vi "Version_2.0_Single_Column_Code.vi"() -> ()   [LabVIEW 2020] (continued)
                                n3037 = call "PortChanger (SubVI).vi"("Port Number"=w3481, "VISA Refnum in"=w3482) -> ()  [unwired: 10 in]
                                }
                                frame #7 {
                                n3038 = local read "VISA Refnum in\nfor Pump"() -> (w3483:refnum<visa-resource-name>)
                                n3039 = call "ProcessCompletionWaiter (SubVI).vi"("VISA Refnum in"=w3483) -> ()  [unwired: 11 in]
                                }
                              }
                            }
                          }
                          frame #3 {
                            # "Wash the pathway between column-2 and column-1 on chip"
                            n3040 = local read "n"() -> (w3484:i32)
                            n3041 = for {
                              N: w3484 -> [_]
                              n3042 = stacked-sequence {
                                frame #0 {
                                n3043 = local read "Buffer-A2 Pumping\nResolution"() -> (w3487:T2)
                                n3044 = local read "VISA Refnum in\nfor Pump"() -> (w3489:refnum<visa-resource-name>)
                                n3045 = local read "V-S"() -> (w3485:dbl)
                                n3046 = local read "Volume of Syringe"() -> (w3488:dbl)
                                n3047 = call "RPickUp(SubVI).vi"("Volume to be picked up"=w3485, "Volume of Syringe"=w3488, "Resolution of PickUP"=w3487, "PickUp Flow Rate (ul/min)"=150.0, "VISA Refnum in"=w3489) -> ()  [unwired: 6 in, 1 out]
                                }
                                frame #1 {
                                n3048 = local read "Stopper that ends \nthe main loops"() -> (w3490:bool)
                                n3049 = local read "VISA Refnum in\nfor Pump"() -> (w3491:refnum<visa-resource-name>)
                                n3050 = case shown="True" w3490 {
                                frame False {
                                }
                                frame True {
                                n3051 = local read "VISA Refnum in\nfor Pump"() -> (w3492:refnum<visa-resource-name>)
                                n3052 = call "HardStopCurrentProcess (SubVI).vi"("VISA Refnum in"=w3492) -> ()  [unwired: 11 in]
                                }
                                }
                                n3053 = call "ProcessCompletionWaiter (SubVI).vi"("VISA Refnum in"=w3491) -> ()  [unwired: 11 in]
                                }
                                frame #2 {
                                # "Switch to Port-10"
                                # "Port-10 of the pump is conncted to column-2"
                                n3054 = local read "VISA Refnum in\nfor Pump"() -> (w3494:refnum<visa-resource-name>)
                                n3055 = call "PortChanger (SubVI).vi"("Port Number"="10", "VISA Refnum in"=w3494) -> ()  [unwired: 10 in]
                                }
                                frame #3 {
                                n3056 = local read "Stopper that ends \nthe main loops"() -> (w3495:bool)
                                n3057 = local read "VISA Refnum in\nfor Pump"() -> (w3496:refnum<visa-resource-name>)
                                n3058 = case shown="True" w3495 {
                                frame False {
                                }
                                frame True {
                                n3059 = local read "VISA Refnum in\nfor Pump"() -> (w3497:refnum<visa-resource-name>)
                                n3060 = call "HardStopCurrentProcess (SubVI).vi"("VISA Refnum in"=w3497) -> ()  [unwired: 11 in]
                                }
                                }
                                n3061 = call "ProcessCompletionWaiter (SubVI).vi"("VISA Refnum in"=w3496) -> ()  [unwired: 11 in]
                                }
                                frame #4 {
                                n3062 = local read "Buffer-A2 Pumping\nResolution"() -> (w3506:T2)
                                n3063 = local read "VISA Refnum in\nfor Pump"() -> (w3508:refnum<visa-resource-name>)
                                n3064 = local read "f"() -> (w3498:dbl)
                                n3065 = local read "Volume of Syringe"() -> (w3507:dbl)
                                n3066 = call "GoToAbsolutePosition(SubVI).vi"("Absolute Volume Position in Syringe (in ul)"=0.0 ("Volume to be Dispensed"), "Volume of Syringe"=w3507, "Resolution of Pumping"=w3506, "Flow Rate (ul/min)"=w3498, "VISA Refnum in"=w3508) -> ()  [unwired: 6 in, 1 out]
                                n3067 = local read "VISA Refnum in\nfor Valve"() -> (w3500:refnum<visa-resource-name>)
                                n3068 = local read "External Valve \nOPEN"() -> (w3499:string)
                                n3069 = local write "Valve V2 Open"(TRUE ("Valve V2 Open")) -> ()
                                n3070 = local write "Valve V1 Open"(FALSE ("Valve V1 Open")) -> ()
                                n3071 = local write "Valve V4 Open"(FALSE ("Valve V4 Open")) -> ()
                                n3072 = local write "Valve V3 Open"(TRUE ("Valve V3 Open")) -> ()
                                n3073 = call "PortChanger_Valve (SubVI).vi"("Port Number"=w3499, "VISA Refnum in"=w3500) -> ()  [unwired: 10 in]
                                }
                                frame #5 {
                                n3074 = local read "VISA Refnum in\nfor Pump"() -> (w3509:refnum<visa-resource-name>)
                                n3075 = call "ProcessCompletionWaiter (SubVI).vi"("VISA Refnum in"=w3509) -> ()  [unwired: 11 in]
                                }
                                frame #6 {
                                # "Change the port back to Buffer-C1"
                                n3076 = local read "VISA Refnum in\nfor Pump"() -> (w3511:refnum<visa-resource-name>)
                                n3077 = local read "Port for \nC1-Equilibriation"() -> (w3510:string)
                                n3078 = call "PortChanger (SubVI).vi"("Port Number"=w3510, "VISA Refnum in"=w3511) -> ()  [unwired: 10 in]
                                }
                                frame #7 {
                                n3079 = local read "VISA Refnum in\nfor Pump"() -> (w3512:refnum<visa-resource-name>)
                                n3080 = call "ProcessCompletionWaiter (SubVI).vi"("VISA Refnum in"=w3512) -> ()  [unwired: 11 in]
                                }
                              }
                            }
                          }
                          frame #4 {
                            # "Washes the SEC column"
                            n3081 = local read "Apparent Volume\nof Syringe"() -> (w3515:dbl)
                            n3082 = local read "c"() -> (w3516:dbl)
                            n3083 = Quotient & Remainder(x=w3516, y=w3515) -> (x-y*floor(x/y)=w3514:dbl, floor(x/y)=w3513:dbl)
                            n3084 = for {
                              N: w3513 -> [_]
                              n3085 = stacked-sequence {
                                frame #0 {
                                n3086 = local read "Buffer-A2 Pumping\nResolution"() -> (w3519:T2)
                                n3087 = local read "VISA Refnum in\nfor Pump"() -> (w3521:refnum<visa-resource-name>)
                                n3088 = local read "Apparent Volume\nof Syringe"() -> (w3517:dbl)
                                n3089 = local read "Volume of Syringe"() -> (w3520:dbl)
                                n3090 = call "RPickUp(SubVI).vi"("Volume to be picked up"=w3517, "Volume of Syringe"=w3520, "Resolution of PickUP"=w3519, "PickUp Flow Rate (ul/min)"=150.0, "VISA Refnum in"=w3521) -> ()  [unwired: 6 in, 1 out]
                                }
                                frame #1 {
                                n3091 = local read "Stopper that ends \nthe main loops"() -> (w3522:bool)
                                n3092 = local read "VISA Refnum in\nfor Pump"() -> (w3523:refnum<visa-resource-name>)
                                n3093 = case shown="True" w3522 {
                                frame False {
                                }
                                frame True {
                                n3094 = local read "VISA Refnum in\nfor Pump"() -> (w3524:refnum<visa-resource-name>)
                                n3095 = call "HardStopCurrentProcess (SubVI).vi"("VISA Refnum in"=w3524) -> ()  [unwired: 11 in]
                                }
                                }
                                n3096 = call "ProcessCompletionWaiter (SubVI).vi"("VISA Refnum in"=w3523) -> ()  [unwired: 11 in]
                                }
                                frame #2 {
                                # "Switch to Port-10"
                                # "Port-10 of the pump is conncted to column-2 of chip"
                                n3097 = local read "VISA Refnum in\nfor Pump"() -> (w3526:refnum<visa-resource-name>)
                                n3098 = call "PortChanger (SubVI).vi"("Port Number"="10", "VISA Refnum in"=w3526) -> ()  [unwired: 10 in]
                                }
                                frame #3 {
                                n3099 = local read "Stopper that ends \nthe main loops"() -> (w3527:bool)
                                n3100 = local read "VISA Refnum in\nfor Pump"() -> (w3528:refnum<visa-resource-name>)
                                n3101 = case shown="True" w3527 {
                                frame False {
                                }
                                frame True {
                                n3102 = local read "VISA Refnum in\nfor Pump"() -> (w3529:refnum<visa-resource-name>)
                                n3103 = call "HardStopCurrentProcess (SubVI).vi"("VISA Refnum in"=w3529) -> ()  [unwired: 11 in]
                                }
                                }
                                n3104 = call "ProcessCompletionWaiter (SubVI).vi"("VISA Refnum in"=w3528) -> ()  [unwired: 11 in]
                                }
                                frame #4 {
                                # "Keeps the AMF valve after column-1 open and valve after column-2 closed"
                                n3105 = local read "Buffer-A2 Pumping\nResolution"() -> (w3541:T2)
                                n3106 = local read "VISA Refnum in\nfor Pump"() -> (w3543:refnum<visa-resource-name>)
                                n3107 = local read "f"() -> (w3533:dbl)
                                n3108 = local write "Valve V3 Open"(FALSE ("Valve V3 Open")) -> ()
                                n3109 = local write "Valve V2 Open"(FALSE ("Valve V2 Open")) -> ()
                                n3110 = local write "Valve V4 Open"(TRUE ("Valve V4 Open")) -> ()
                                n3111 = local write "Valve V1 Open"(FALSE ("Valve V1 Open")) -> ()
                                n3112 = local read "Volume of Syringe"() -> (w3542:dbl)
                                n3113 = call "GoToAbsolutePosition(SubVI).vi"("Absolute Volume Position in Syringe (in ul)"=0.0 ("Volume to be Dispensed"), "Volume of Syringe"=w3542, "Resolution of Pumping"=w3541, "Flow Rate (ul/min)"=w3533, "VISA Refnum in"=w3543) -> ()  [unwired: 6 in, 1 out]
                                n3114 = local read "VISA Refnum in\nfor Valve"() -> (w3538:refnum<visa-resource-name>)
                                n3115 = local read "External Valve \nCLOSED"() -> (w3534:string)
                                n3116 = local write "Valve V5 Open"(TRUE ("Valve V5 Open")) -> ()
                                n3117 = local write "Valve V6 Open"(FALSE ("Valve V6 Open")) -> ()
                                n3118 = local write "Valve V7 Open"(TRUE ("Valve V7 Open")) -> ()
                                n3119 = call "PortChanger_Valve (SubVI).vi"("Port Number"=w3534, "VISA Refnum in"=w3538) -> ()  [unwired: 10 in]
                                }
                                frame #5 {
                                n3120 = local read "VISA Refnum in\nfor Pump"() -> (w3544:refnum<visa-resource-name>)
                                n3121 = call "ProcessCompletionWaiter (SubVI).vi"("VISA Refnum in"=w3544) -> ()  [unwired: 11 in]
                                }
                                frame #6 {
                                # "Change the port back to Buffer-C1"
                                n3122 = local read "VISA Refnum in\nfor Pump"() -> (w3546:refnum<visa-resource-name>)
                                n3123 = local read "Port for \nC1-Equilibriation"() -> (w3545:string)
                                n3124 = call "PortChanger (SubVI).vi"("Port Number"=w3545, "VISA Refnum in"=w3546) -> ()  [unwired: 10 in]
                                }
                                frame #7 {
                                n3125 = local read "VISA Refnum in\nfor Pump"() -> (w3547:refnum<visa-resource-name>)
                                n3126 = call "ProcessCompletionWaiter (SubVI).vi"("VISA Refnum in"=w3547) -> ()  [unwired: 11 in]
                                }
                              }
                            }
                            n3127 = local write "Reminder of the \nVolume to be \nPumped"(w3514) -> ()
                          }
                          frame #5 {
                            # "Washes the SEC column"
                            n3128 = stacked-sequence {
                              frame #0 {
                                n3129 = local read "Buffer-A2 Pumping\nResolution"() -> (w3550:T2)
                                n3130 = local read "VISA Refnum in\nfor Pump"() -> (w3552:refnum<visa-resource-name>)
                                n3131 = local read "Reminder of the \nVolume to be \nPumped"() -> (w3548:dbl)
                                n3132 = local read "Volume of Syringe"() -> (w3551:dbl)
                                n3133 = call "RPickUp(SubVI).vi"("Volume to be picked up"=w3548, "Volume of Syringe"=w3551, "Resolution of PickUP"=w3550, "PickUp Flow Rate (ul/min)"=150.0, "VISA Refnum in"=w3552) -> ()  [unwired: 6 in, 1 out]
                              }
                              frame #1 {
                                n3134 = local read "Stopper that ends \nthe main loops"() -> (w3553:bool)
                                n3135 = local read "VISA Refnum in\nfor Pump"() -> (w3554:refnum<visa-resource-name>)
                                n3136 = case shown="True" w3553 {
                                frame False {
                                }
                                frame True {
                                n3137 = local read "VISA Refnum in\nfor Pump"() -> (w3555:refnum<visa-resource-name>)
                                n3138 = call "HardStopCurrentProcess (SubVI).vi"("VISA Refnum in"=w3555) -> ()  [unwired: 11 in]
                                }
                                }
                                n3139 = call "ProcessCompletionWaiter (SubVI).vi"("VISA Refnum in"=w3554) -> ()  [unwired: 11 in]
                              }
                              frame #2 {
                                # "Switch to Port-10"
                                # "Port-10 of the pump is conncted to column-2 of chip"
                                n3140 = local read "VISA Refnum in\nfor Pump"() -> (w3557:refnum<visa-resource-name>)
                                n3141 = call "PortChanger (SubVI).vi"("Port Number"="10", "VISA Refnum in"=w3557) -> ()  [unwired: 10 in]
                              }
                              frame #3 {
                                n3142 = local read "Stopper that ends \nthe main loops"() -> (w3558:bool)
                                n3143 = local read "VISA Refnum in\nfor Pump"() -> (w3559:refnum<visa-resource-name>)
                                n3144 = case shown="True" w3558 {
                                frame False {
                                }
                                frame True {
                                n3145 = local read "VISA Refnum in\nfor Pump"() -> (w3560:refnum<visa-resource-name>)
                                n3146 = call "HardStopCurrentProcess (SubVI).vi"("VISA Refnum in"=w3560) -> ()  [unwired: 11 in]
                                }
                                }
                                n3147 = call "ProcessCompletionWaiter (SubVI).vi"("VISA Refnum in"=w3559) -> ()  [unwired: 11 in]
                              }
                              frame #4 {
                                n3148 = local read "Buffer-A2 Pumping\nResolution"() -> (w3572:T2)
                                n3149 = local read "VISA Refnum in\nfor Pump"() -> (w3574:refnum<visa-resource-name>)
                                n3150 = local read "f"() -> (w3564:dbl)
                                n3151 = local read "Volume of Syringe"() -> (w3573:dbl)
                                n3152 = call "GoToAbsolutePosition(SubVI).vi"("Absolute Volume Position in Syringe (in ul)"=0.0 ("Volume to be Dispensed"), "Volume of Syringe"=w3573, "Resolution of Pumping"=w3572, "Flow Rate (ul/min)"=w3564, "VISA Refnum in"=w3574) -> ()  [unwired: 6 in, 1 out]
                                n3153 = local write "Valve V3 Open"(FALSE ("Valve V3 Open")) -> ()
                                n3154 = local write "Valve V2 Open"(FALSE ("Valve V2 Open")) -> ()
                                n3155 = local write "Valve V1 Open"(FALSE ("Valve V1 Open")) -> ()
                                n3156 = local write "Valve V4 Open"(TRUE ("Valve V4 Open")) -> ()
                                n3157 = local read "VISA Refnum in\nfor Valve"() -> (w3569:refnum<visa-resource-name>)
                                n3158 = local read "External Valve \nCLOSED"() -> (w3565:string)
                                n3159 = local write "Valve V6 Open"(TRUE ("Valve V6 Open")) -> ()
                                n3160 = local write "Valve V5 Open"(TRUE ("Valve V5 Open")) -> ()
                                n3161 = local write "Valve V7 Open"(TRUE ("Valve V7 Open")) -> ()
                                n3162 = call "PortChanger_Valve (SubVI).vi"("Port Number"=w3565, "VISA Refnum in"=w3569) -> ()  [unwired: 10 in]
                              }
                              frame #5 {
                                n3163 = local read "VISA Refnum in\nfor Pump"() -> (w3575:refnum<visa-resource-name>)
                                n3164 = call "ProcessCompletionWaiter (SubVI).vi"("VISA Refnum in"=w3575) -> ()  [unwired: 11 in]
                              }
                            }
                          }
                        }
                        n3165 = local write "Washing Column-1"(FALSE ("Washing Column-1")) -> ()
                        n3166 = local write "Washing Column-2"(TRUE ("Washing Column-2")) -> ()
                      }
                      frame #4 {
                        # "Elute Column-1, Divert Sample into Column-2, Elute column-2 and Divert the sample onto Grid"
                        n3167 = stacked-sequence {
                          frame #0 {
                            # "Switch to Port-7"
                            # "Port-7 of pump is connected to Buffer-B"
                            n3168 = local write "Washing Column-2"(FALSE ("Washing Column-2")) -> ()
                            n3169 = local read "VISA Refnum in\nfor Pump"() -> (w3580:refnum<visa-resource-name>)
                            n3170 = local read "Port for \nB-Elution"() -> (w3578:string)
                            n3171 = local write "Affinity Elution On"(TRUE ("Affinity Elution On")) -> ()
                            n3172 = call "PortChanger (SubVI).vi"("Port Number"=w3578, "VISA Refnum in"=w3580) -> ()  [unwired: 10 in]
                            n3173 = local write "Elution of Column-1"(TRUE ("Elution of Column-1")) -> ()
                          }
                          frame #1 {
                            n3174 = local read "VISA Refnum in\nfor Pump"() -> (w3581:refnum<visa-resource-name>)
                            n3175 = call "ProcessCompletionWaiter (SubVI).vi"("VISA Refnum in"=w3581) -> ()  [unwired: 11 in]
                          }
                          frame #2 {
                            # "If Yes, it will clean the elution buffer from port-5 tubing a bit more"
                            n3176 = local read "Clean the \nBuffer-B tubing"() -> (w3582:bool)
                            n3177 = case shown="True" w3582 {
                              frame False {
                                n3178 = stacked-sequence {
                                frame #0 {
                                n3179 = local read "Buffer-B Pumping\nResolution"() -> (w3585:T2)
                                n3180 = local read "VISA Refnum in\nfor Pump"() -> (w3587:refnum<visa-resource-name>)
                                n3181 = local read "V-S"() -> (w3584:dbl)
                                n3182 = local read "Volume of Syringe"() -> (w3586:dbl)
                                n3183 = call "RPickUp(SubVI).vi"("Volume to be picked up"=w3584, "Volume of Syringe"=w3586, "Resolution of PickUP"=w3585, "PickUp Flow Rate (ul/min)"=150.0, "VISA Refnum in"=w3587) -> ()  [unwired: 6 in, 1 out]
                                }
                                frame #1 {
                                n3184 = local read "Stopper that ends \nthe main loops"() -> (w3588:bool)
                                n3185 = local read "VISA Refnum in\nfor Pump"() -> (w3589:refnum<visa-resource-name>)
                                n3186 = case shown="True" w3588 {
                                frame False {
                                }
                                frame True {
                                n3187 = local read "VISA Refnum in\nfor Pump"() -> (w3590:refnum<visa-resource-name>)
                                n3188 = call "HardStopCurrentProcess (SubVI).vi"("VISA Refnum in"=w3590) -> ()  [unwired: 11 in]
                                }
                                }
                                n3189 = call "ProcessCompletionWaiter (SubVI).vi"("VISA Refnum in"=w3589) -> ()  [unwired: 11 in]
                                }
                                frame #2 {
                                n3190 = local read "VISA Refnum in\nfor Pump"() -> (w3592:refnum<visa-resource-name>)
                                n3191 = call "PortChanger (SubVI).vi"("Port Number"="1", "VISA Refnum in"=w3592) -> ()  [unwired: 10 in]
                                }
                                frame #3 {
                                n3192 = local read "Stopper that ends \nthe main loops"() -> (w3593:bool)
                                n3193 = local read "VISA Refnum in\nfor Pump"() -> (w3594:refnum<visa-resource-name>)
                                n3194 = case shown="True" w3593 {
                                frame False {
                                }
                                frame True {
                                n3195 = local read "VISA Refnum in\nfor Pump"() -> (w3595:refnum<visa-resource-name>)
                                n3196 = call "HardStopCurrentProcess (SubVI).vi"("VISA Refnum in"=w3595) -> ()  [unwired: 11 in]
                                }
                                }
                                n3197 = call "ProcessCompletionWaiter (SubVI).vi"("VISA Refnum in"=w3594) -> ()  [unwired: 11 in]
                                }
                                frame #4 {
                                n3198 = local read "VISA Refnum in\nfor Pump"() -> (w3600:refnum<visa-resource-name>)
                                n3199 = local read "Volume of Syringe"() -> (w3597:dbl)
                                n3200 = call "GoToAbsolutePosition(SubVI).vi"("Absolute Volume Position in Syringe (in ul)"=0.0, "Volume of Syringe"=w3597, "Resolution of Pumping"=T2."Standard Pumping", "Flow Rate (ul/min)"=150.0, "VISA Refnum in"=w3600) -> ()  [unwired: 6 in, 1 out]
                                }
                                frame #5 {
                                n3201 = local read "Stopper that ends \nthe main loops"() -> (w3601:bool)
                                n3202 = local read "VISA Refnum in\nfor Pump"() -> (w3602:refnum<visa-resource-name>)
                                n3203 = case shown="True" w3601 {
                                frame False {
                                }
                                frame True {
                                n3204 = local read "VISA Refnum in\nfor Pump"() -> (w3603:refnum<visa-resource-name>)
                                n3205 = call "HardStopCurrentProcess (SubVI).vi"("VISA Refnum in"=w3603) -> ()  [unwired: 11 in]
                                }
                                }
                                n3206 = call "ProcessCompletionWaiter (SubVI).vi"("VISA Refnum in"=w3602) -> ()  [unwired: 11 in]
                                }
                                }
                              }
                              frame True {
                                n3207 = for {
                                N: 2 -> [_]
                                n3208 = stacked-sequence {
                                frame #0 {
                                n3209 = local read "Buffer-B Pumping\nResolution"() -> (w3607:T2)
                                n3210 = local read "VISA Refnum in\nfor Pump"() -> (w3609:refnum<visa-resource-name>)
                                n3211 = local read "Apparent Volume\nof Syringe"() -> (w3606:dbl)
                                n3212 = local read "Volume of Syringe"() -> (w3608:dbl)
                                n3213 = call "RPickUp(SubVI).vi"("Volume to be picked up"=w3606, "Volume of Syringe"=w3608, "Resolution of PickUP"=w3607, "PickUp Flow Rate (ul/min)"=150.0, "VISA Refnum in"=w3609) -> ()  [unwired: 6 in, 1 out]
                                }
                                frame #1 {
                                n3214 = local read "Stopper that ends \nthe main loops"() -> (w3610:bool)
                                n3215 = local read "VISA Refnum in\nfor Pump"() -> (w3611:refnum<visa-resource-name>)
                                n3216 = case shown="True" w3610 {
                                frame False {
                                }
                                frame True {
                                n3217 = local read "VISA Refnum in\nfor Pump"() -> (w3612:refnum<visa-resource-name>)
                                n3218 = call "HardStopCurrentProcess (SubVI).vi"("VISA Refnum in"=w3612) -> ()  [unwired: 11 in]
                                }
                                }
                                n3219 = call "ProcessCompletionWaiter (SubVI).vi"("VISA Refnum in"=w3611) -> ()  [unwired: 11 in]
                                }
                                frame #2 {
                                n3220 = local read "VISA Refnum in\nfor Pump"() -> (w3614:refnum<visa-resource-name>)
                                n3221 = call "PortChanger (SubVI).vi"("Port Number"="1", "VISA Refnum in"=w3614) -> ()  [unwired: 10 in]
                                }
                                frame #3 {
                                n3222 = local read "Stopper that ends \nthe main loops"() -> (w3615:bool)
                                n3223 = local read "VISA Refnum in\nfor Pump"() -> (w3616:refnum<visa-resource-name>)
                                n3224 = case shown="True" w3615 {
                                frame False {
                                }
                                frame True {
                                n3225 = local read "VISA Refnum in\nfor Pump"() -> (w3617:refnum<visa-resource-name>)
                                n3226 = call "HardStopCurrentProcess (SubVI).vi"("VISA Refnum in"=w3617) -> ()  [unwired: 11 in]
                                }
                                }
                                n3227 = call "ProcessCompletionWaiter (SubVI).vi"("VISA Refnum in"=w3616) -> ()  [unwired: 11 in]
                                }
                                frame #4 {
                                n3228 = local read "VISA Refnum in\nfor Pump"() -> (w3622:refnum<visa-resource-name>)
                                n3229 = local read "Volume of Syringe"() -> (w3619:dbl)
                                n3230 = call "GoToAbsolutePosition(SubVI).vi"("Absolute Volume Position in Syringe (in ul)"=0.0, "Volume of Syringe"=w3619, "Resolution of Pumping"=T2."Standard Pumping", "Flow Rate (ul/min)"=150.0, "VISA Refnum in"=w3622) -> ()  [unwired: 6 in, 1 out]
                                }
                                frame #5 {
                                n3231 = local read "Stopper that ends \nthe main loops"() -> (w3623:bool)
                                n3232 = local read "VISA Refnum in\nfor Pump"() -> (w3624:refnum<visa-resource-name>)
                                n3233 = case shown="True" w3623 {
                                frame False {
                                }
                                frame True {
                                n3234 = local read "VISA Refnum in\nfor Pump"() -> (w3625:refnum<visa-resource-name>)
                                n3235 = call "HardStopCurrentProcess (SubVI).vi"("VISA Refnum in"=w3625) -> ()  [unwired: 11 in]
                                }
                                }
                                n3236 = call "ProcessCompletionWaiter (SubVI).vi"("VISA Refnum in"=w3624) -> ()  [unwired: 11 in]
                                }
                                }
                                }
                              }
                            }
                          }
                          frame #3 {
                            n3237 = local read "VISA Refnum in\nfor Pump"() -> (w3627:refnum<visa-resource-name>)
                            n3238 = local read "Port for \nB-Elution"() -> (w3626:string)
                            n3239 = call "PortChanger (SubVI).vi"("Port Number"=w3626, "VISA Refnum in"=w3627) -> ()  [unwired: 10 in]
                          }
                          frame #4 {
                            n3240 = local read "VISA Refnum in\nfor Pump"() -> (w3628:refnum<visa-resource-name>)
                            n3241 = call "ProcessCompletionWaiter (SubVI).vi"("VISA Refnum in"=w3628) -> ()  [unwired: 11 in]
                          }
                          frame #5 {
                            n3242 = local read "Buffer-B PickUp \nFlow Rate (ul/min)"() -> (w3631:dbl)
                            n3243 = local read "Buffer-B Pumping\nResolution"() -> (w3630:T2)
                            n3244 = local read "VISA Refnum in\nfor Pump"() -> (w3633:refnum<visa-resource-name>)
                            n3245 = local read "Buffer-B Volume \nto be  Pumped"() -> (w3629:dbl)
                            n3246 = local read "Volume of Syringe"() -> (w3632:dbl)
                            n3247 = call "RPickUp(SubVI).vi"("Volume to be picked up"=w3629, "Volume of Syringe"=w3632, "Resolution of PickUP"=w3630, "PickUp Flow Rate (ul/min)"=w3631, "VISA Refnum in"=w3633) -> ()  [unwired: 6 in, 1 out]
                          }
                          frame #6 {
                            n3248 = local read "Stopper that ends \nthe main loops"() -> (w3634:bool)
                            n3249 = local read "VISA Refnum in\nfor Pump"() -> (w3635:refnum<visa-resource-name>)
                            n3250 = case shown="True" w3634 {
                              frame False {
                              }
                              frame True {
                                n3251 = local read "VISA Refnum in\nfor Pump"() -> (w3636:refnum<visa-resource-name>)
                                n3252 = call "HardStopCurrentProcess (SubVI).vi"("VISA Refnum in"=w3636) -> ()  [unwired: 11 in]
                              }
                            }
                            n3253 = call "ProcessCompletionWaiter (SubVI).vi"("VISA Refnum in"=w3635) -> ()  [unwired: 11 in]
                          }
                          frame #7 {
                            # "Reads the initial Plunger Position for computing the volume dispensed"
                            n3254 = local read "VISA Refnum in\nfor Pump"() -> (w3638:refnum<visa-resource-name>)
                            n3255 = call "AbsolutePlungerPosition (SubVI).vi"("VISA Refnum in"=w3638) -> ("Plunger Position"=w3637:i32)  [unwired: 10 in]
                            n3256 = local write "Initial Plunger Position"(w3637) -> ()
                          }
                          frame #8 {
                            # "Switch to Port-2"
                            # "Port-2 of the pump is conncted to column-1 of chip"
                            n3257 = local read "VISA Refnum in\nfor Pump"() -> (w3640:refnum<visa-resource-name>)
                            n3258 = call "PortChanger (SubVI).vi"("Port Number"="2", "VISA Refnum in"=w3640) -> ()  [unwired: 10 in]
                          }
                          frame #9 {
                            n3259 = local read "Stopper that ends \nthe main loops"() -> (w3641:bool)
                            n3260 = local read "VISA Refnum in\nfor Pump"() -> (w3642:refnum<visa-resource-name>)
                            n3261 = case shown="True" w3641 {
                              frame False {
                              }
                              frame True {
                                n3262 = local read "VISA Refnum in\nfor Pump"() -> (w3643:refnum<visa-resource-name>)
                                n3263 = call "HardStopCurrentProcess (SubVI).vi"("VISA Refnum in"=w3643) -> ()  [unwired: 11 in]
                              }
                            }
                            n3264 = call "ProcessCompletionWaiter (SubVI).vi"("VISA Refnum in"=w3642) -> ()  [unwired: 11 in]
                          }
                          frame #10 {
                            # "Keeps the AMF valve after column-1 open and valve after column-2 closed"
                            n3265 = local read "VISA Refnum in\nfor Valve"() -> (w3648:refnum<visa-resource-name>)
                            n3266 = local read "External Valve \nOPEN"() -> (w3647:string)
                            n3267 = call "PortChanger_Valve (SubVI).vi"("Port Number"=w3647, "VISA Refnum in"=w3648) -> ()  [unwired: 10 in]
                            n3268 = local write "Valve V1 Open"(TRUE ("Valve V1 Open")) -> ()
                            n3269 = local write "Valve V2 Open"(TRUE ("Valve V2 Open")) -> ()
                            n3270 = local write "Valve V3 Open"(FALSE ("Valve V3 Open")) -> ()
                            n3271 = local write "Valve V4 Open"(FALSE ("Valve V4 Open")) -> ()
                            n3272 = local write "Valve V6 Open"(FALSE ("Valve V6 Open")) -> ()
                            n3273 = local write "Valve V5 Open"(FALSE ("Valve V5 Open")) -> ()
                            n3274 = local write "Valve V7 Open"(FALSE ("Valve V7 Open")) -> ()
                          }
                          frame #11 {
                            n3275 = local read "Buffer-B Dispense\nFlow Rate (ul/min)"() -> (w3658:dbl)
                            n3276 = local read "Buffer-B Pumping\nResolution"() -> (w3657:T2)
                            n3277 = local read "Initial Plunger Position"() -> (w3654:dbl)
                            n3278 = local read "VISA Refnum in\nfor Pump"() -> (w3660:refnum<visa-resource-name>)
                            n3279 = local read "Volume of Syringe"() -> (w3659:dbl)
                            n3280 = call "GoToAbsolutePosition(SubVI).vi"("Absolute Volume Position in Syringe (in ul)"=0.0 ("Volume to be Dispensed"), "Volume of Syringe"=w3659, "Resolution of Pumping"=w3657, "Flow Rate (ul/min)"=w3658, "VISA Refnum in"=w3660) -> ()  [unwired: 6 in, 1 out]
                            n3281 = local write "Pause Data Collection"(FALSE ("Pause Data Collection")) -> ()
                            n3282 = local write "Vol_now"(0.0 ("Vol_now")) -> ()
                            n3283 = local write "Position\nNow"(w3654) -> ()
                          }
                          frame #12 {
                            n3284 = while {
                              stop <- w3667 stop-if-true
                              n3285 = event shown="[0] \"Pause Elution Value\": Value Change" {
                                selector: _ -> [_ _]
                                dyn-events: _ -> [_ _]
                                timeout: 100 -> [_ _]
                                event "Pause Elution\nValue": Value Change {
                                n3286 = event-data() -> ()  [unwired: 1 in, 6 out]
                                n3287 = stacked-sequence {
                                frame #0 {
                                n3288 = local read "Pause Elution"() -> (w3669:bool)
                                n3289 = case shown="False" w3669 {
                                frame False {
                                n3290 = local write "Pause Elution"(TRUE ("Pause Elution")) -> ()
                                }
                                frame True {
                                n3291 = local write "Pause Elution"(FALSE ("Pause Elution")) -> ()
                                }
                                }
                                }
                                frame #1 {
                                n3292 = local read "Pause Elution"() -> (w3672:bool)
                                n3293 = case shown="False" w3672 {
                                frame False {
                                n3294 = local read "Buffer-B Dispense\nFlow Rate (ul/min)"() -> (w3677:dbl)
                                n3295 = local read "VISA Refnum in\nfor Pump"() -> (w3678:refnum<visa-resource-name>)
                                n3296 = local read "Buffer-B Pumping\nResolution"() -> (w3674:T2)
                                n3297 = local read "Volume of Syringe"() -> (w3675:dbl)
                                n3298 = call "GoToAbsolutePosition(SubVI).vi"("Absolute Volume Position in Syringe (in ul)"=0.0, "Volume of Syringe"=w3675, "Resolution of Pumping"=w3674, "Flow Rate (ul/min)"=w3677, "VISA Refnum in"=w3678) -> ()  [unwired: 6 in, 1 out]
                                n3299 = local write "Pause Data Collection"(FALSE ("Pause Data Collection")) -> ()
                                }
                                frame True {
                                n3300 = local read "VISA Refnum in\nfor Pump"() -> (w3680:refnum<visa-resource-name>)
                                n3301 = local write "Pause Data Collection"(TRUE ("Pause Data Collection")) -> ()
                                n3302 = call "HardStopCurrentProcess (SubVI).vi"("VISA Refnum in"=w3680) -> ()  [unwired: 11 in]
                                }
                                }
                                }
                                }
                                }
                                event Timeout {
                                n3303 = event-data() -> ()  [unwired: 1 in, 3 out]
                                }
                              }
                              n3304 = local read "Divert Sample \ninto Column-2"() -> (w3666:bool)
                              n3305 = local read "Stopper that ends \nthe main loops"() -> (w3665:bool)
                              n3306 = Or(x=w3666, y=w3665) -> (x .or. y?=w3667:bool)
                            }
                            n3307 = local read "Buffer-B Pumping\nResolution"() -> (w3663:T2)
                            n3308 = local read "VISA Refnum in\nfor Pump"() -> (w3664:refnum<visa-resource-name>)
                            n3309 = local read "Volume of Syringe"() -> (w3662:dbl)
                            n3310 = while {
                              tunnel: w3664 -> [w3689]
                              tunnel: w3663 -> [w3688]
                              tunnel: w3662 -> [w3687]
                              stop <- w3683 stop-if-true
                              n3311 = local read "Position\nNow"() -> (w3681:dbl)
                              n3312 = local read "Pause Elution"() -> (w3682:bool)
                              n3313 = case shown="True" w3682 {
                                tunnel: w3681 -> [w3693 _]
                                tunnel: w3689 -> [w3692 w3735]
                                tunnel: w3688 -> [w3691 _]
                                tunnel: w3687 -> [w3690 _]
                                frame False {
                                n3314 = stacked-sequence {
                                tunnel: w3693 -> [_ w3699]
                                tunnel: w3692 -> [_ w3698]
                                tunnel: w3691 -> [_ w3697]
                                tunnel: w3690 -> [_ w3696]
                                frame #0 {
                                n3315 = Wait (ms)(milliseconds to wait=u32 3000) -> ()  [unwired: 1 out]
                                n3316 = local write "Signal"(TRUE ("Signal")) -> ()
                                }
                                frame #1 {
                                n3317 = while {
                                tunnel: w3699 -> [w3711]
                                tunnel: w3698 -> [w3710]
                                tunnel: w3697 -> [w3709]
                                tunnel: w3696 -> [w3708]
                                stop <- w3703 stop-if-true
                                n3318 = stacked-sequence {
                                tunnel: w3711 -> [_ w3718]
                                tunnel: w3710 -> [_ w3717]
                                tunnel: w3709 -> [_ w3716]
                                tunnel: w3708 -> [_ w3715]
                                frame #0 {
                                n3319 = Wait (ms)(milliseconds to wait=u32 500) -> ()  [unwired: 1 out]
                                }
                                frame #1 {
                                n3320 = call "AbsolutePlungerPosition (SubVI).vi"("VISA Refnum in"=w3717) -> ("Plunger Position"=w3714:i32)  [unwired: 10 in]
                                n3321 = case shown="\"High Resolution Pumping\"" w3716 {
                                tunnel: w3718 -> [w3723 w3732]
                                tunnel: w3714 -> [w3724 w3731]
                                tunnel: [w3722 w3729] -> w3713
                                tunnel: w3715 -> [w3721 w3730]
                                frame "Standard Pumping", Default {
                                n3322 = Subtract(x=w3723, y=w3724) -> (x-y=w3720:dbl)
                                n3323 = Absolute Value(x=w3720) -> (abs(x)=w3719:dbl)
                                n3324 = Multiply(x=w3719, y=w3721) -> (x*y=w3726:dbl)
                                n3325 = Divide(x=w3726, y=3000.0) -> (x/y=w3722:dbl)
                                }
                                frame "High Resolution Pumping" {
                                n3326 = Subtract(x=w3732, y=w3731) -> (x-y=w3728:dbl)
                                n3327 = Absolute Value(x=w3728) -> (abs(x)=w3727:dbl)
                                n3328 = Multiply(x=w3727, y=w3730) -> (x*y=w3734:dbl)
                                n3329 = Divide(x=w3734, y=24000.0) -> (x/y=w3729:dbl)
                                }
                                }
                                n3330 = local write "Volume being Injected \nin this process"(w3713) -> ()
                                }
                                }
                                n3331 = local read "Volume being Injected \nin this process"() -> (w3701:dbl)
                                n3332 = local read "Affinity Elution \nGraph Min CutOff"() -> (w3700:dbl)
                                n3333 = local read "Stopper that ends \nthe main loops"() -> (w3706:bool)
                                n3334 = local read "Divert Sample \ninto Column-2"() -> (w3707:bool)
                                n3335 = Greater Or Equal?(x=w3701, y=w3700) -> (x >= y?=w3702:bool)
                                n3336 = Or(x=w3707, y=w3706) -> (x .or. y?=w3704:bool)
                                n3337 = local read "Pause Elution"() -> (w3705:bool)
                                n3338 = local write "Affinity Elution \nis Approaching"(w3702) -> ()
                                n3339 = Or(x=w3705, y=w3704) -> (x .or. y?=w3703:bool)
                                }
                                }
                                }
                                }
                                frame True {
                                n3340 = stacked-sequence {
                                tunnel: w3735 -> [_ w3738 _]
                                frame #0 {
                                n3341 = Wait (ms)(milliseconds to wait=u32 2000) -> ()  [unwired: 1 out]
                                }
                                frame #1 {
                                n3342 = local read "Signal"() -> (w3737:bool)
                                n3343 = case shown="True" w3737 {
                                tunnel: w3738 -> [_ w3744]
                                frame False {
                                }
                                frame True {
                                n3344 = local read "Volume being Injected \nin this process"() -> (w3742:dbl)
                                n3345 = local read "Net Elution \nVolume"() -> (w3741:dbl)
                                n3346 = local write "Signal"(FALSE ("Signal")) -> ()
                                n3347 = Add(x=w3742, y=w3741) -> (x+y=w3740:dbl)
                                n3348 = call "AbsolutePlungerPosition (SubVI).vi"("VISA Refnum in"=w3744) -> ("Plunger Position"=w3743:i32)  [unwired: 10 in]
                                n3349 = local write "Net Elution \nVolume"(w3740) -> ()
                                n3350 = local write "Position\nNow"(w3743) -> ()
                                }
                                }
                                }
                                frame #2 {
                                n3351 = local write "Volume being Injected \nin this process"(0.0 ("Volume being Injected \nin this process")) -> ()
                                }
                                }
                                }
                              }
                              n3352 = local read "Stopper that ends \nthe main loops"() -> (w3685:bool)
                              n3353 = local read "Divert Sample \ninto Column-2"() -> (w3684:bool)
                              n3354 = Or(x=w3684, y=w3685) -> (x .or. y?=w3683:bool)
                              n3355 = Wait (ms)(milliseconds to wait=u32 300) -> ()  [unwired: 1 out]
                            }
                            n3356 = local read "Stopper that ends \nthe main loops"() -> (w3661:bool)
                            n3357 = case shown="True" w3661 {
                              frame False {
                              }
                              frame True {
                                n3358 = local read "VISA Refnum in\nfor Pump"() -> (w3746:refnum<visa-resource-name>)
                                n3359 = call "HardStopCurrentProcess (SubVI).vi"("VISA Refnum in"=w3746) -> ()  [unwired: 11 in]
                              }
                            }
                          }
                          frame #13 {
                            # "valve after column-1 is closed"
                            # "Keeps the on-chip Valve V1 and V3 after column-2 open"
                            # "Keeps the AMF valve after column-1 closed and valve after column-2 open"
                            n3360 = local read "VISA Refnum in\nfor Pump"() -> (w3759:refnum<visa-resource-name>)
                            n3361 = local read "Volume being Injected \nin this process"() -> (w3756:dbl)
                            n3362 = local write "Sample Volume Diverted\ninto Column-2"(0.0 ("Sample Volume Diverted\ninto Column-2")) -> ()
                            n3363 = call "AbsolutePlungerPosition (SubVI).vi"("VISA Refnum in"=w3759) -> ("Plunger Position"=w3758:i32)  [unwired: 10 in]
                            n3364 = local write "Position\nNow"(w3758) -> ()
                            n3365 = local write "Vol_previous"(0.0 ("Vol_diff")) -> ()
                            n3366 = local write "Vol_now"(w3756) -> ()
                            n3367 = local read "VISA Refnum in\nfor Valve"() -> (w3751:refnum<visa-resource-name>)
                            n3368 = local read "External Valve \nCLOSED"() -> (w3750:string)
                            n3369 = local write "Valve V1 Open"(TRUE ("Valve V1 Open")) -> ()
                            n3370 = local write "Valve V3 Open"(TRUE ("Valve V3 Open")) -> ()
                            n3371 = local write "Valve V2 Open"(FALSE ("Valve V2 Open")) -> ()
                            n3372 = local write "Valve V4 Open"(TRUE ("Valve V4 Open")) -> ()
                            n3373 = call "PortChanger_Valve (SubVI).vi"("Port Number"=w3750, "VISA Refnum in"=w3751) -> ()  [unwired: 10 in]
                            n3374 = local write "Valve V5 Open"(TRUE ("Valve V5 Open")) -> ()
                            n3375 = local write "Valve V6 Open"(FALSE ("Valve V6 Open")) -> ()
                            n3376 = local write "Valve V7 Open"(TRUE ("Valve V7 Open")) -> ()
                          }
                          frame #14 {
                            n3377 = local read "Divert Sample \ninto Column-2"() -> (w3761:bool)
                            n3378 = case shown="True" w3761 {
                              frame False {
                                n3379 = stacked-sequence {
                                frame #0 {
                                n3380 = local read "Buffer-B Pumping\nResolution"() -> (w3764:T2)
                                n3381 = local read "VISA Refnum in\nfor Pump"() -> (w3766:refnum<visa-resource-name>)
                                n3382 = local read "Initial Plunger Position"() -> (w3765:dbl)
                                n3383 = local read "Volume of Syringe"() -> (w3763:dbl)
                                n3384 = while {
                                tunnel: w3765 -> [w3772]
                                tunnel: w3766 -> [w3771]
                                tunnel: w3764 -> [w3770]
                                tunnel: w3763 -> [w3769]
                                stop <- w3767 stop-if-true
                                n3385 = Wait (ms)(milliseconds to wait=u32 100) -> ()  [unwired: 1 out]
                                n3386 = stacked-sequence {
                                tunnel: w3772 -> [w3778 _]
                                tunnel: w3771 -> [w3777 w3798]
                                tunnel: w3770 -> [w3776 _]
                                tunnel: w3769 -> [w3775 _]
                                tunnel: [_ w3796] -> w3767
                                frame #0 {
                                n3387 = call "AbsolutePlungerPosition (SubVI).vi"("VISA Refnum in"=w3777) -> ("Plunger Position"=w3774:i32)  [unwired: 10 in]
                                n3388 = case shown="\"Standard Pumping\", Default" w3776 {
                                tunnel: w3778 -> [w3783 w3792]
                                tunnel: w3774 -> [w3784 w3791]
                                tunnel: [w3782 w3789] -> w3773
                                tunnel: w3775 -> [w3781 w3790]
                                frame "Standard Pumping", Default {
                                n3389 = Subtract(x=w3783, y=w3784) -> (x-y=w3780:dbl)
                                n3390 = Absolute Value(x=w3780) -> (abs(x)=w3779:dbl)
                                n3391 = Multiply(x=w3779, y=w3781) -> (x*y=w3786:dbl)
                                n3392 = Divide(x=w3786, y=3000.0) -> (x/y=w3782:dbl)
                                }
                                frame "High Resolution Pumping" {
                                n3393 = Subtract(x=w3792, y=w3791) -> (x-y=w3788:dbl)
                                n3394 = Absolute Value(x=w3788) -> (abs(x)=w3787:dbl)
                                n3395 = Multiply(x=w3787, y=w3790) -> (x*y=w3794:dbl)
                                n3396 = Divide(x=w3794, y=24000.0) -> (x/y=w3789:dbl)
                                }
                                }
                                n3397 = local write "Volume being Injected \nin this process"(w3773) -> ()
                                }
                                frame #1 {
                                n3398 = local read "Stopper that ends \nthe main loops"() -> (w3795:bool)
                                n3399 = call "LSPOneStatus (SubVI).vi"("VISA Refnum in"=w3798) -> ("read buffer"=w3800:string)  [unwired: 10 in]
                                n3400 = call <vilib>:"Trim Whitespace.vi"("string"=w3800) -> ("trimmed string"=w3799:string)  [unwired: 1 in]
                                n3401 = Equal?(x=w3799, y="/0`\u0003") -> (x = y?=w3797:bool)
                                n3402 = Or(x=w3797, y=w3795) -> (x .or. y?=w3796:bool)
                                }
                                }
                                }
                                n3403 = local read "Stopper that ends \nthe main loops"() -> (w3762:bool)
                                n3404 = case shown="True" w3762 {
                                frame False {
                                }
                                frame True {
                                n3405 = local read "VISA Refnum in\nfor Pump"() -> (w3802:refnum<visa-resource-name>)
                                n3406 = call "HardStopCurrentProcess (SubVI).vi"("VISA Refnum in"=w3802) -> ()  [unwired: 11 in]
                                }
                                }
                                }
                                }
                              }
                              frame True {
                                n3407 = stacked-sequence {
                                frame #0 {
                                n3408 = local read "Buffer-B Pumping\nResolution"() -> (w3805:T2)
                                n3409 = local read "VISA Refnum in\nfor Pump"() -> (w3807:refnum<visa-resource-name>)
                                n3410 = local read "Volume of Syringe"() -> (w3804:dbl)
                                n3411 = local read "Position\nNow"() -> (w3806:dbl)
                                n3412 = while {
                                tunnel: w3806 -> [w3813]
                                tunnel: w3807 -> [w3812]
                                tunnel: w3805 -> [w3811]
                                tunnel: w3804 -> [w3810]
                                stop <- w3808 stop-if-true
                                n3413 = Wait (ms)(milliseconds to wait=u32 100) -> ()  [unwired: 1 out]
                                n3414 = stacked-sequence {
                                tunnel: w3813 -> [w3823 _ _]
                                tunnel: w3812 -> [w3822 _ w3849]
                                tunnel: w3811 -> [w3821 _ _]
                                tunnel: w3810 -> [w3820 _ _]
                                tunnel: [_ _ w3847] -> w3808
                                frame #0 {
                                n3415 = local read "Vol_previous"() -> (w3817:dbl)
                                n3416 = call "AbsolutePlungerPosition (SubVI).vi"("VISA Refnum in"=w3822) -> ("Plunger Position"=w3819:i32)  [unwired: 10 in]
                                n3417 = case shown="\"Standard Pumping\", Default" w3821 {
                                tunnel: w3823 -> [w3828 w3837]
                                tunnel: w3819 -> [w3829 w3836]
                                tunnel: [w3827 w3834] -> w3818
                                tunnel: w3820 -> [w3826 w3835]
                                frame "Standard Pumping", Default {
                                n3418 = Subtract(x=w3828, y=w3829) -> (x-y=w3825:dbl)
                                n3419 = Absolute Value(x=w3825) -> (abs(x)=w3824:dbl)
                                n3420 = Multiply(x=w3824, y=w3826) -> (x*y=w3831:dbl)
                                n3421 = Divide(x=w3831, y=3000.0) -> (x/y=w3827:dbl)
                                }
                                frame "High Resolution Pumping" {
                                n3422 = Subtract(x=w3837, y=w3836) -> (x-y=w3833:dbl)
                                n3423 = Absolute Value(x=w3833) -> (abs(x)=w3832:dbl)
                                n3424 = Multiply(x=w3832, y=w3835) -> (x*y=w3839:dbl)
                                n3425 = Divide(x=w3839, y=24000.0) -> (x/y=w3834:dbl)
                                }
                                }
                                n3426 = Subtract(x=w3818, y=w3817) -> (x-y=w3816:dbl)
                                n3427 = local read "Vol_now"() -> (w3814:dbl)
                                n3428 = local write "Sample Volume Diverted\ninto Column-2"(w3818) -> ()
                                n3429 = Add(x=w3816, y=w3814) -> (x+y=w3815:dbl)
                                n3430 = local write "Volume being Injected \nin this process"(w3815) -> ()
                                }
                                frame #1 {
                                n3431 = local read "Volume being Injected \nin this process"() -> (w3840:dbl)
                                n3432 = local read "Sample Volume Diverted\ninto Column-2"() -> (w3841:dbl)
                                n3433 = local write "Vol_now"(w3840) -> ()
                                n3434 = local write "Vol_previous"(w3841) -> ()
                                }
                                frame #2 {
                                n3435 = local read "Buffer-B Volume \nto be Pumped for\nSample Diversion\nto Column-2"() -> (w3843:dbl)
                                n3436 = local read "Sample Volume Diverted\ninto Column-2"() -> (w3842:dbl)
                                n3437 = local read "Stopper that ends \nthe main loops"() -> (w3844:bool)
                                n3438 = call "LSPOneStatus (SubVI).vi"("VISA Refnum in"=w3849) -> ("read buffer"=w3851:string)  [unwired: 10 in]
                                n3439 = call <vilib>:"Trim Whitespace.vi"("string"=w3851) -> ("trimmed string"=w3850:string)  [unwired: 1 in]
                                n3440 = Equal?(x=w3850, y="/0`\u0003") -> (x = y?=w3848:bool)
                                n3441 = Greater Or Equal?(x=w3842, y=w3843) -> (x >= y?=w3846:bool)
                                n3442 = Or(x=w3844, y=w3846) -> (x .or. y?=w3845:bool)
                                n3443 = Or(x=w3848, y=w3845) -> (x .or. y?=w3847:bool)
                                }
                                }
                                }
                                n3444 = local read "Stopper that ends \nthe main loops"() -> (w3803:bool)
                                n3445 = case shown="True" w3803 {
                                frame False {
                                }
                                frame True {
                                n3446 = local read "VISA Refnum in\nfor Pump"() -> (w3853:refnum<visa-resource-name>)
                                n3447 = call "HardStopCurrentProcess (SubVI).vi"("VISA Refnum in"=w3853) -> ()  [unwired: 11 in]
                                }
                                }
                                }
                                frame #1 {
                                n3448 = local read "VISA Refnum in\nfor Pump"() -> (w3855:refnum<visa-resource-name>)
                                n3449 = local write "Pause Data Collection"(TRUE ("Pause Data Collection")) -> ()
                                n3450 = call "HardStopCurrentProcess (SubVI).vi"("VISA Refnum in"=w3855) -> ()  [unwired: 11 in]
                                }
                                frame #2 {
                                n3451 = local read "VISA Refnum in\nfor Pump"() -> (w3856:refnum<visa-resource-name>)
                                n3452 = call "PortChanger (SubVI).vi"("Port Number"="1", "VISA Refnum in"=w3856) -> ()  [unwired: 10 in]
                                }
                                frame #3 {
                                n3453 = local read "VISA Refnum in\nfor Pump"() -> (w3862:refnum<visa-resource-name>)
                                n3454 = local read "Volume of Syringe"() -> (w3858:dbl)
                                n3455 = call "GoToAbsolutePosition(SubVI).vi"("Absolute Volume Position in Syringe (in ul)"=0.0, "Volume of Syringe"=w3858, "Resolution of Pumping"=T2."Standard Pumping", "Flow Rate (ul/min)"=150.0, "VISA Refnum in"=w3862) -> ()  [unwired: 6 in, 1 out]
                                }
                                frame #4 {
                                n3456 = local read "VISA Refnum in\nfor Pump"() -> (w3864:refnum<visa-resource-name>)
                                n3457 = local write "Divert Sample \ninto Column-2"(FALSE ("Divert Sample \ninto Column-2")) -> ()
                                n3458 = call "ProcessCompletionWaiter (SubVI).vi"("VISA Refnum in"=w3864) -> ()  [unwired: 11 in]
                                }
                                }
                              }
                            }
                          }
                          frame #15 {
                            # "Keeps the On-Chip Valves V1 and V3 closed"
                            # "Switch to Port-5/8"
                            # "Port-5/8 of pump is connected to Buffer-C1/C2"
                            # "Keeps the AMF valve after column-1 open and valve after column-2 closed"
                            n3459 = local read "VISA Refnum in\nfor Pump"() -> (w3877:refnum<visa-resource-name>)
                            n3460 = local write "Pause Data Collection"(TRUE ("Pause Data Collection")) -> ()
                            n3461 = Wait (ms)(milliseconds to wait=u32 500) -> ()  [unwired: 1 out]
                            n3462 = local write "Affinity On"(FALSE ("Affinity On")) -> ()
                            n3463 = local read "Port for \nC2-Elution"() -> (w3868:string)
                            n3464 = local write "Affinity Elution On"(FALSE ("Affinity Elution On")) -> ()
                            n3465 = call "PortChanger (SubVI).vi"("Port Number"=w3868, "VISA Refnum in"=w3877) -> ()  [unwired: 10 in]
                            n3466 = local read "VISA Refnum in\nfor Valve"() -> (w3871:refnum<visa-resource-name>)
                            n3467 = local read "External Valve \nCLOSED"() -> (w3870:string)
                            n3468 = local write "Valve V1 Open"(FALSE ("Valve V1 Open")) -> ()
                            n3469 = local write "Valve V2 Open"(FALSE ("Valve V2 Open")) -> ()
                            n3470 = local write "Valve V3 Open"(FALSE ("Valve V3 Open")) -> ()
                            n3471 = local write "Valve V4 Open"(FALSE ("Valve V4 Open")) -> ()
                            n3472 = call "PortChanger_Valve (SubVI).vi"("Port Number"=w3870, "VISA Refnum in"=w3871) -> ()  [unwired: 10 in]
                            n3473 = local write "Valve V5 Open"(FALSE ("Valve V5 Open")) -> ()
                            n3474 = local write "Valve V6 Open"(FALSE ("Valve V6 Open")) -> ()
                            n3475 = local write "Valve V7 Open"(FALSE ("Valve V7 Open")) -> ()
                          }
                          frame #16 {
                            n3476 = local read "VISA Refnum in\nfor Pump"() -> (w3881:refnum<visa-resource-name>)
                            n3477 = call "ProcessCompletionWaiter (SubVI).vi"("VISA Refnum in"=w3881) -> ()  [unwired: 11 in]
                            n3478 = local write "Start the Process"(FALSE ("Start the Process")) -> ()
                          }
                          frame #17 {
                            n3479 = local read "Stopper that ends \nthe main loops"() -> (w3885:bool)
                            n3480 = local read "Start the Process"() -> (w3886:bool)
                            n3481 = Or(x=w3886, y=w3885) -> (x .or. y?=w3884:bool)
                            n3482 = local write "Elution of Column-1"(FALSE ("Elution of Column-1")) -> ()
                            n3483 = case shown="False" w3884 {
                              frame False {
                                n3484 = while {
                                stop <- w3890 stop-if-true
                                n3485 = local read "Stopper that ends \nthe main loops"() -> (w3891:bool)
                                n3486 = local read "Start the Process"() -> (w3892:bool)
                                n3487 = Or(x=w3892, y=w3891) -> (x .or. y?=w3890:bool)
                                n3488 = Wait (ms)(milliseconds to wait=u32 10) -> ()  [unwired: 1 out]
                                }
                                n3489 = One Button Dialog(message="Move to Column-2 detection zone and Press 'Start the Process' Button.") -> ()  [unwired: 1 in, 1 out]
                              }
                              frame True {
                              }
                            }
                            n3490 = local write "Volume being Injected \nin this process"(0.0 ("Volume being Injected \nin this process")) -> ()
                            n3491 = local write "Elution of Column-2"(TRUE ("Elution of Column-2")) -> ()
                          }
                          frame #18 {
                            # "If Yes, it will clean the SEC buffer from port-8 tubing else it will clean the pump valve a bit"
                            n3492 = local read "Clean the \nBuffer-C2 tubing"() -> (w3893:bool)
                            n3493 = case shown="False" w3893 {
                              frame False {
                                n3494 = stacked-sequence {
                                frame #0 {
                                n3495 = local read "VISA Refnum in\nfor Pump"() -> (w3895:refnum<visa-resource-name>)
                                n3496 = local read "Port for \nC2-Elution"() -> (w3894:string)
                                n3497 = call "PortChanger (SubVI).vi"("Port Number"=w3894, "VISA Refnum in"=w3895) -> ()  [unwired: 10 in]
                                }
                                frame #1 {
                                n3498 = local read "VISA Refnum in\nfor Pump"() -> (w3896:refnum<visa-resource-name>)
                                n3499 = call "ProcessCompletionWaiter (SubVI).vi"("VISA Refnum in"=w3896) -> ()  [unwired: 11 in]
                                }
                                frame #2 {
                                n3500 = local read "Buffer-C2 Pumping\nResolution"() -> (w3899:T2)
                                n3501 = local read "VISA Refnum in\nfor Pump"() -> (w3901:refnum<visa-resource-name>)
                                n3502 = local read "V-S"() -> (w3897:dbl)
                                n3503 = local read "Volume of Syringe"() -> (w3900:dbl)
                                n3504 = call "RPickUp(SubVI).vi"("Volume to be picked up"=w3897, "Volume of Syringe"=w3900, "Resolution of PickUP"=w3899, "PickUp Flow Rate (ul/min)"=150.0, "VISA Refnum in"=w3901) -> ()  [unwired: 6 in, 1 out]
                                }
                                frame #3 {
                                n3505 = local read "Stopper that ends \nthe main loops"() -> (w3902:bool)
                                n3506 = local read "VISA Refnum in\nfor Pump"() -> (w3903:refnum<visa-resource-name>)
                                n3507 = case shown="True" w3902 {
                                frame False {
                                }
                                frame True {
                                n3508 = local read "VISA Refnum in\nfor Pump"() -> (w3904:refnum<visa-resource-name>)
                                n3509 = call "HardStopCurrentProcess (SubVI).vi"("VISA Refnum in"=w3904) -> ()  [unwired: 11 in]
                                }
                                }
                                n3510 = call "ProcessCompletionWaiter (SubVI).vi"("VISA Refnum in"=w3903) -> ()  [unwired: 11 in]
                                }
                                frame #4 {
                                n3511 = local read "VISA Refnum in\nfor Pump"() -> (w3906:refnum<visa-resource-name>)
                                n3512 = call "PortChanger (SubVI).vi"("Port Number"="1", "VISA Refnum in"=w3906) -> ()  [unwired: 10 in]
                                }
                                frame #5 {
                                n3513 = local read "Stopper that ends \nthe main loops"() -> (w3907:bool)
                                n3514 = local read "VISA Refnum in\nfor Pump"() -> (w3908:refnum<visa-resource-name>)
                                n3515 = case shown="True" w3907 {
                                frame False {
                                }
                                frame True {
                                n3516 = local read "VISA Refnum in\nfor Pump"() -> (w3909:refnum<visa-resource-name>)
                                n3517 = call "HardStopCurrentProcess (SubVI).vi"("VISA Refnum in"=w3909) -> ()  [unwired: 11 in]
                                }
                                }
                                n3518 = call "ProcessCompletionWaiter (SubVI).vi"("VISA Refnum in"=w3908) -> ()  [unwired: 11 in]
                                }
                                frame #6 {
                                n3519 = local read "VISA Refnum in\nfor Pump"() -> (w3914:refnum<visa-resource-name>)
                                n3520 = local read "Volume of Syringe"() -> (w3911:dbl)
                                n3521 = call "GoToAbsolutePosition(SubVI).vi"("Absolute Volume Position in Syringe (in ul)"=0.0, "Volume of Syringe"=w3911, "Resolution of Pumping"=T2."Standard Pumping", "Flow Rate (ul/min)"=150.0, "VISA Refnum in"=w3914) -> ()  [unwired: 6 in, 1 out]
                                }
                                frame #7 {
                                n3522 = local read "Stopper that ends \nthe main loops"() -> (w3915:bool)
                                n3523 = local read "VISA Refnum in\nfor Pump"() -> (w3916:refnum<visa-resource-name>)
                                n3524 = case shown="True" w3915 {
                                frame False {
                                }
                                frame True {
                                n3525 = local read "VISA Refnum in\nfor Pump"() -> (w3917:refnum<visa-resource-name>)
                                n3526 = call "HardStopCurrentProcess (SubVI).vi"("VISA Refnum in"=w3917) -> ()  [unwired: 11 in]
                                }
                                }
                                n3527 = call "ProcessCompletionWaiter (SubVI).vi"("VISA Refnum in"=w3916) -> ()  [unwired: 11 in]
                                }
                                }
                              }
                              frame True {
                                n3528 = for {
                                N: 2 -> [_]
                                n3529 = stacked-sequence {
                                frame #0 {
                                n3530 = local read "VISA Refnum in\nfor Pump"() -> (w3920:refnum<visa-resource-name>)
                                n3531 = local read "Port for \nC2-Elution"() -> (w3919:string)
                                n3532 = call "PortChanger (SubVI).vi"("Port Number"=w3919, "VISA Refnum in"=w3920) -> ()  [unwired: 10 in]
                                }
                                frame #1 {
                                n3533 = local read "VISA Refnum in\nfor Pump"() -> (w3921:refnum<visa-resource-name>)
                                n3534 = call "ProcessCompletionWaiter (SubVI).vi"("VISA Refnum in"=w3921) -> ()  [unwired: 11 in]
                                }
                                frame #2 {
                                n3535 = local read "Buffer-C2 Pumping\nResolution"() -> (w3924:T2)
                                n3536 = local read "VISA Refnum in\nfor Pump"() -> (w3926:refnum<visa-resource-name>)
                                n3537 = local read "Apparent Volume\nof Syringe"() -> (w3922:dbl)
                                n3538 = local read "Volume of Syringe"() -> (w3925:dbl)
                                n3539 = call "RPickUp(SubVI).vi"("Volume to be picked up"=w3922, "Volume of Syringe"=w3925, "Resolution of PickUP"=w3924, "PickUp Flow Rate (ul/min)"=150.0, "VISA Refnum in"=w3926) -> ()  [unwired: 6 in, 1 out]
                                }
                                frame #3 {
                                n3540 = local read "Stopper that ends \nthe main loops"() -> (w3927:bool)
                                n3541 = local read "VISA Refnum in\nfor Pump"() -> (w3928:refnum<visa-resource-name>)
                                n3542 = case shown="True" w3927 {
                                frame False {
                                }
                                frame True {
                                n3543 = local read "VISA Refnum in\nfor Pump"() -> (w3929:refnum<visa-resource-name>)
                                n3544 = call "HardStopCurrentProcess (SubVI).vi"("VISA Refnum in"=w3929) -> ()  [unwired: 11 in]
                                }
                                }
                                n3545 = call "ProcessCompletionWaiter (SubVI).vi"("VISA Refnum in"=w3928) -> ()  [unwired: 11 in]
                                }
                                frame #4 {
                                n3546 = local read "VISA Refnum in\nfor Pump"() -> (w3931:refnum<visa-resource-name>)
                                n3547 = call "PortChanger (SubVI).vi"("Port Number"="1", "VISA Refnum in"=w3931) -> ()  [unwired: 10 in]
                                }
                                frame #5 {
                                n3548 = local read "Stopper that ends \nthe main loops"() -> (w3932:bool)
                                n3549 = local read "VISA Refnum in\nfor Pump"() -> (w3933:refnum<visa-resource-name>)
                                n3550 = case shown="True" w3932 {
                                frame False {
                                }
                                frame True {
                                n3551 = local read "VISA Refnum in\nfor Pump"() -> (w3934:refnum<visa-resource-name>)
                                n3552 = call "HardStopCurrentProcess (SubVI).vi"("VISA Refnum in"=w3934) -> ()  [unwired: 11 in]
                                }
                                }
                                n3553 = call "ProcessCompletionWaiter (SubVI).vi"("VISA Refnum in"=w3933) -> ()  [unwired: 11 in]
                                }
                                frame #6 {
                                n3554 = local read "VISA Refnum in\nfor Pump"() -> (w3939:refnum<visa-resource-name>)
                                n3555 = local read "Volume of Syringe"() -> (w3936:dbl)
                                n3556 = call "GoToAbsolutePosition(SubVI).vi"("Absolute Volume Position in Syringe (in ul)"=0.0, "Volume of Syringe"=w3936, "Resolution of Pumping"=T2."Standard Pumping", "Flow Rate (ul/min)"=150.0, "VISA Refnum in"=w3939) -> ()  [unwired: 6 in, 1 out]
                                }
                                frame #7 {
                                n3557 = local read "Stopper that ends \nthe main loops"() -> (w3940:bool)
                                n3558 = local read "VISA Refnum in\nfor Pump"() -> (w3941:refnum<visa-resource-name>)
                                n3559 = case shown="True" w3940 {
                                frame False {
                                }
                                frame True {
                                n3560 = local read "VISA Refnum in\nfor Pump"() -> (w3942:refnum<visa-resource-name>)
                                n3561 = call "HardStopCurrentProcess (SubVI).vi"("VISA Refnum in"=w3942) -> ()  [unwired: 11 in]
                                }
                                }
                                n3562 = call "ProcessCompletionWaiter (SubVI).vi"("VISA Refnum in"=w3941) -> ()  [unwired: 11 in]
                                }
                                }
                                }
                              }
                            }
                          }
                          frame #19 {
                            n3563 = local read "VISA Refnum in\nfor Pump"() -> (w3944:refnum<visa-resource-name>)
                            n3564 = local read "Port for \nC2-Elution"() -> (w3943:string)
                            n3565 = call "PortChanger (SubVI).vi"("Port Number"=w3943, "VISA Refnum in"=w3944) -> ()  [unwired: 10 in]
                          }
                          frame #20 {
                            n3566 = local read "VISA Refnum in\nfor Pump"() -> (w3945:refnum<visa-resource-name>)
                            n3567 = call "ProcessCompletionWaiter (SubVI).vi"("VISA Refnum in"=w3945) -> ()  [unwired: 11 in]
                          }
                          frame #21 {
                            n3568 = local read "Buffer-C2 PickUp \nFlow Rate (ul/min)"() -> (w3949:dbl)
                            n3569 = local read "Buffer-C2 Pumping\nResolution"() -> (w3948:T2)
